vi "writeSpreadsheetFile.vi"() -> ()   [LabVIEW 2014]
uses:
  <vilib>/Utility/file.llb/Write To Spreadsheet File (string).vi
panel:
  out "Set?":bool
  in  "stop":bool
  in  "Add":bool
  in  "file path (dialog if empty)":path
  in  "Array":string[](array[string])
  # "Constant Name"
  # "Constant Value"
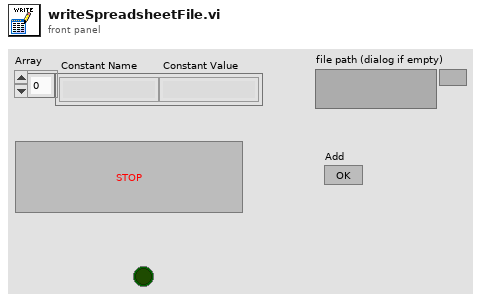
[diagram p1: front panel]
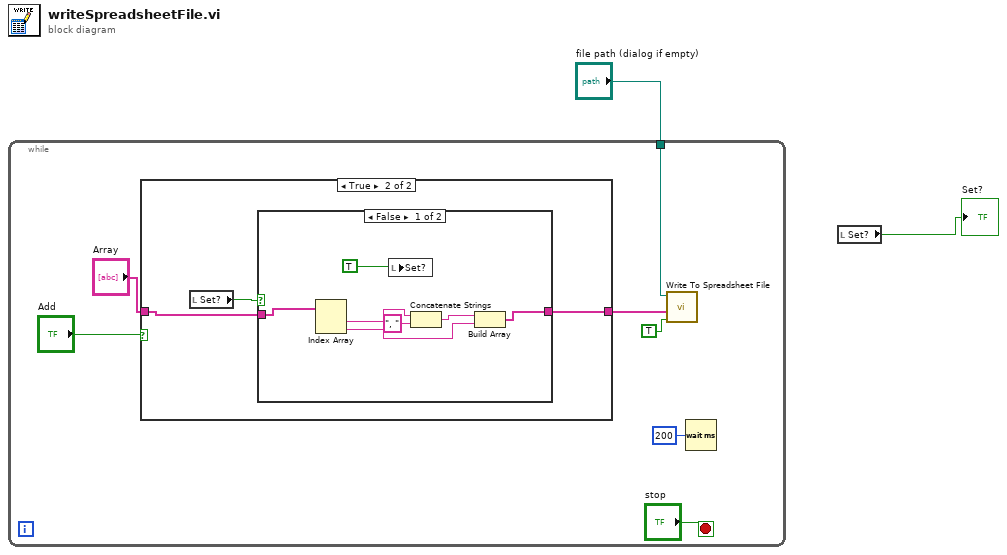
[diagram p0: block diagram]
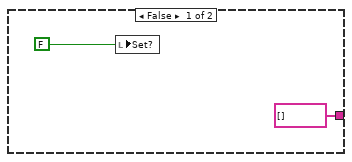
[diagram p2: hidden frame]
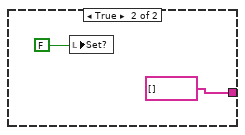
[diagram p3: hidden frame]
diagram:
  n1 = while {
    tunnel: "file path (dialog if empty)" -> [w7]
    stop <- "stop" stop-if-true
    n2 = case shown="True" "Add" {
      tunnel: [string[] [] ("Array") w13] -> w3
      tunnel: "Array" -> [_ w12]
      frame False {
        n3 = local write "Set?"(FALSE) -> ()
      }
      frame True {
        n4 = local read "Set?"() -> (w14:bool)
        n5 = case shown="False" w14 {
          tunnel: [w15 string[] [] ("Array")] -> w13
          tunnel: w12 -> [w20 _]
          frame False {
            n6 = Index Array(array=w20) -> (element #1=w18:string, element #2=w16:string)  [unwired: 2 in]
            n7 = local write "Set?"(TRUE) -> ()
            n8 = Concatenate Strings(w18, ", " ("string")) -> (w17:string)
            n9 = Build Array(w17, w16) -> (w15:string[])
          }
          frame True {
            n10 = local write "Set?"(FALSE) -> ()
          }
        }
      }
    }
    n11 = call-poly <vilib>:"Write To Spreadsheet File.vi"("append to file? (new file:F)"=TRUE, "1D data"=w3, "file path (dialog if empty)"=w7) -> ()  [unwired: 5 in, 1 out]
    n12 = Wait (ms)(milliseconds to wait=u32 200) -> ()  [unwired: 1 out]
  }
  n13 = local read "Set?"() -> (→"Set?":bool)
